vi "4_9.vi"() -> ()   [LabVIEW 2020]
panel:
  out "Numb of \"z\"":i32
  in  "word":string
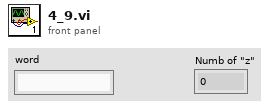
[diagram p1: front panel]
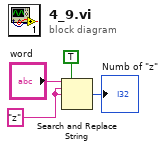
[diagram p0: block diagram]
diagram:
  w3 = "z"
  n1 = Search and Replace String(replace all?=TRUE, input string="word", search string=w3, replace string=w3) -> (number of replacements=→"Numb of \"z\"":i32)  [unwired: 4 in, 3 out]
